vi "pulse Tx 8 spc.vi"(8 "clear DDS":bool, 9 "enable line":bool=TRUE, 10 "take it!":bool, 11 "Cluster":T2={"PW"=0, "frequency shift"=0.0, "amp"=0.9999923706054688, "mode type"=enum."CW", "mode depth"=0, "mode filter"=0, "phase shift"=0.0, "pulse shape filter"=0, "sub spc delay"=0}) -> (0 "output valid":bool, 1 "IQ out":T1[](array[typedef]), 2 "free dds":bool, 4 "frequncy":fxp<+/-,48,0>, 6 "phase":fxp<+/-,16,1>)   [LabVIEW 2021]
uses:
  pulse_tx_vis/pdw.ctl
  pulse_tx_vis/CTL/mode_type.ctl
  <instrlib>/_niInstr/DSP/v1/Shared/Public/IQ Data.ctl
  <instrlib>/_niInstr/DSP/v1/FPGA/Public/Sub VIs/Frequency Shift/Frequency Shift - 8 spc.vi
  <instrlib>/_niInstr/Basic Elements/v1/FPGA/Private/Count Up U32.vi
  <vilib>/rvi/FXPMathLib/FxpAdd/XNode/nifxpmath_Add.xnode
  <instrlib>/_niInstr/DSP/v1/Shared/niInstr DSP v1 Shared.lvlib
  <instrlib>/_niInstr/Basic Elements/v1/FPGA/niInstr Basic Elements v1 FPGA.lvlib
  <vilib>/rvi/FXPMathLib/sim/FxpSim.dll
  <instrlib>/_niInstr/DSP/v1/FPGA/niInstr DSP v1 FPGA.lvlib
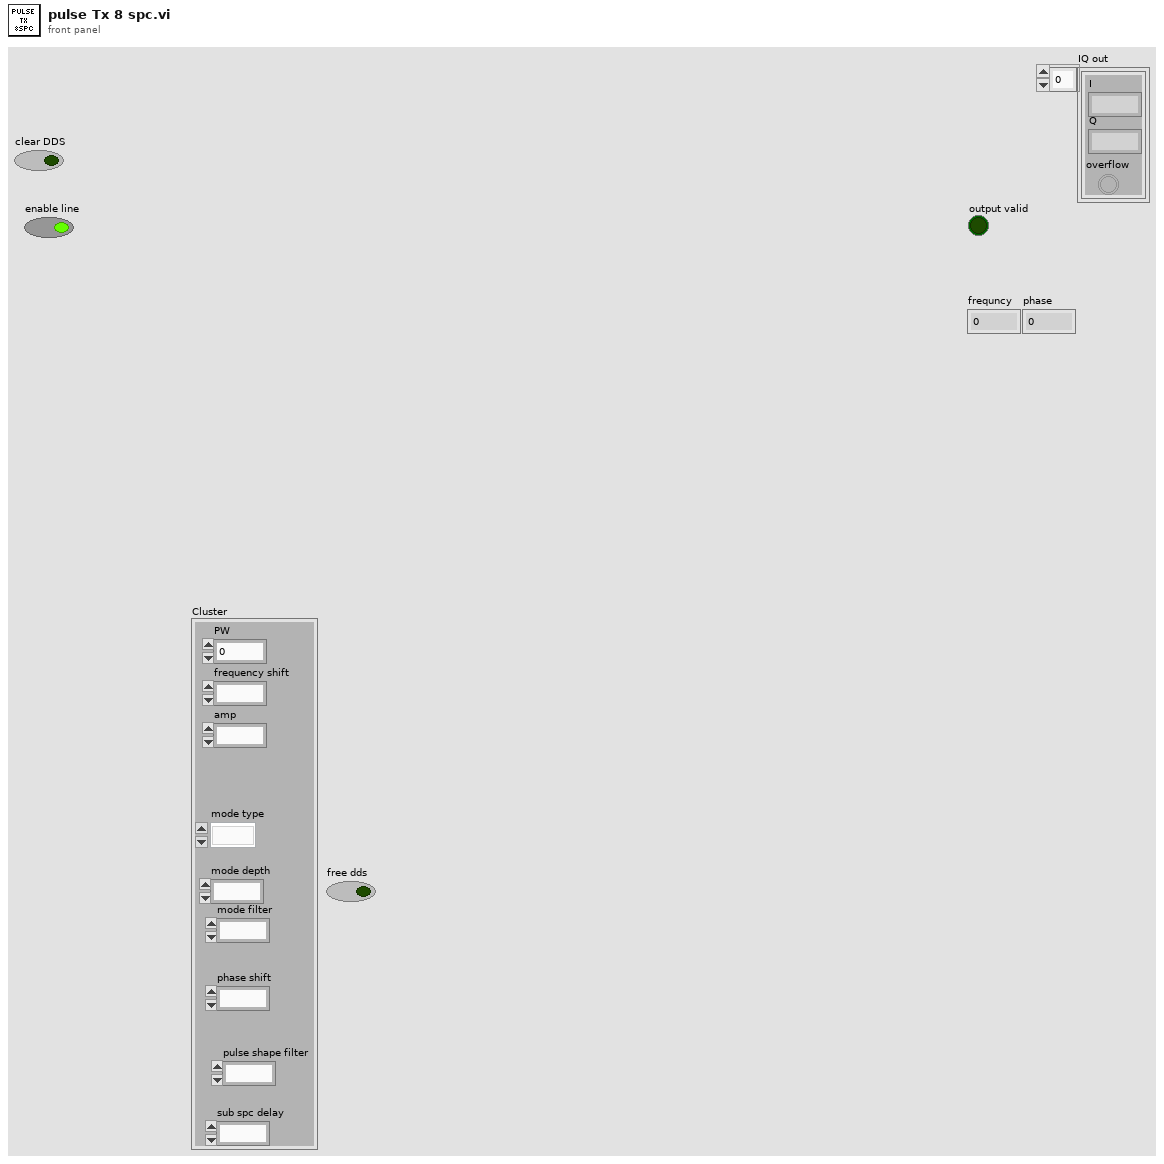
[diagram p1: front panel]
types:
  T1 = typedef "niInstr DSP v1 Shared.lvlib/IQ Data.ctl" = cluster{"I":fxp<+/-,18,1>, "Q":fxp<+/-,18,1>, "overflow":bool}
  T2 = typedef "pdw.ctl" = cluster{"PW":u32, "frequency shift":fxp<+/-,48,0>, "amp":fxp<+/-,18,1>, "mode type":T3, "mode depth":u32, "mode filter":u8, "phase shift":fxp<+/-,16,1>, "pulse shape filter":u8, "sub spc delay":u8}
  T3 = typedef "mode_type.ctl" = enum8{"CW", "from memory 1", "NC - cw", "LFM", "BPSK", "QPSK"}
  T4 = cluster{"I":fxp<+/-,18,1>, "Q":fxp<+/-,18,1>, "overflow":bool}[]
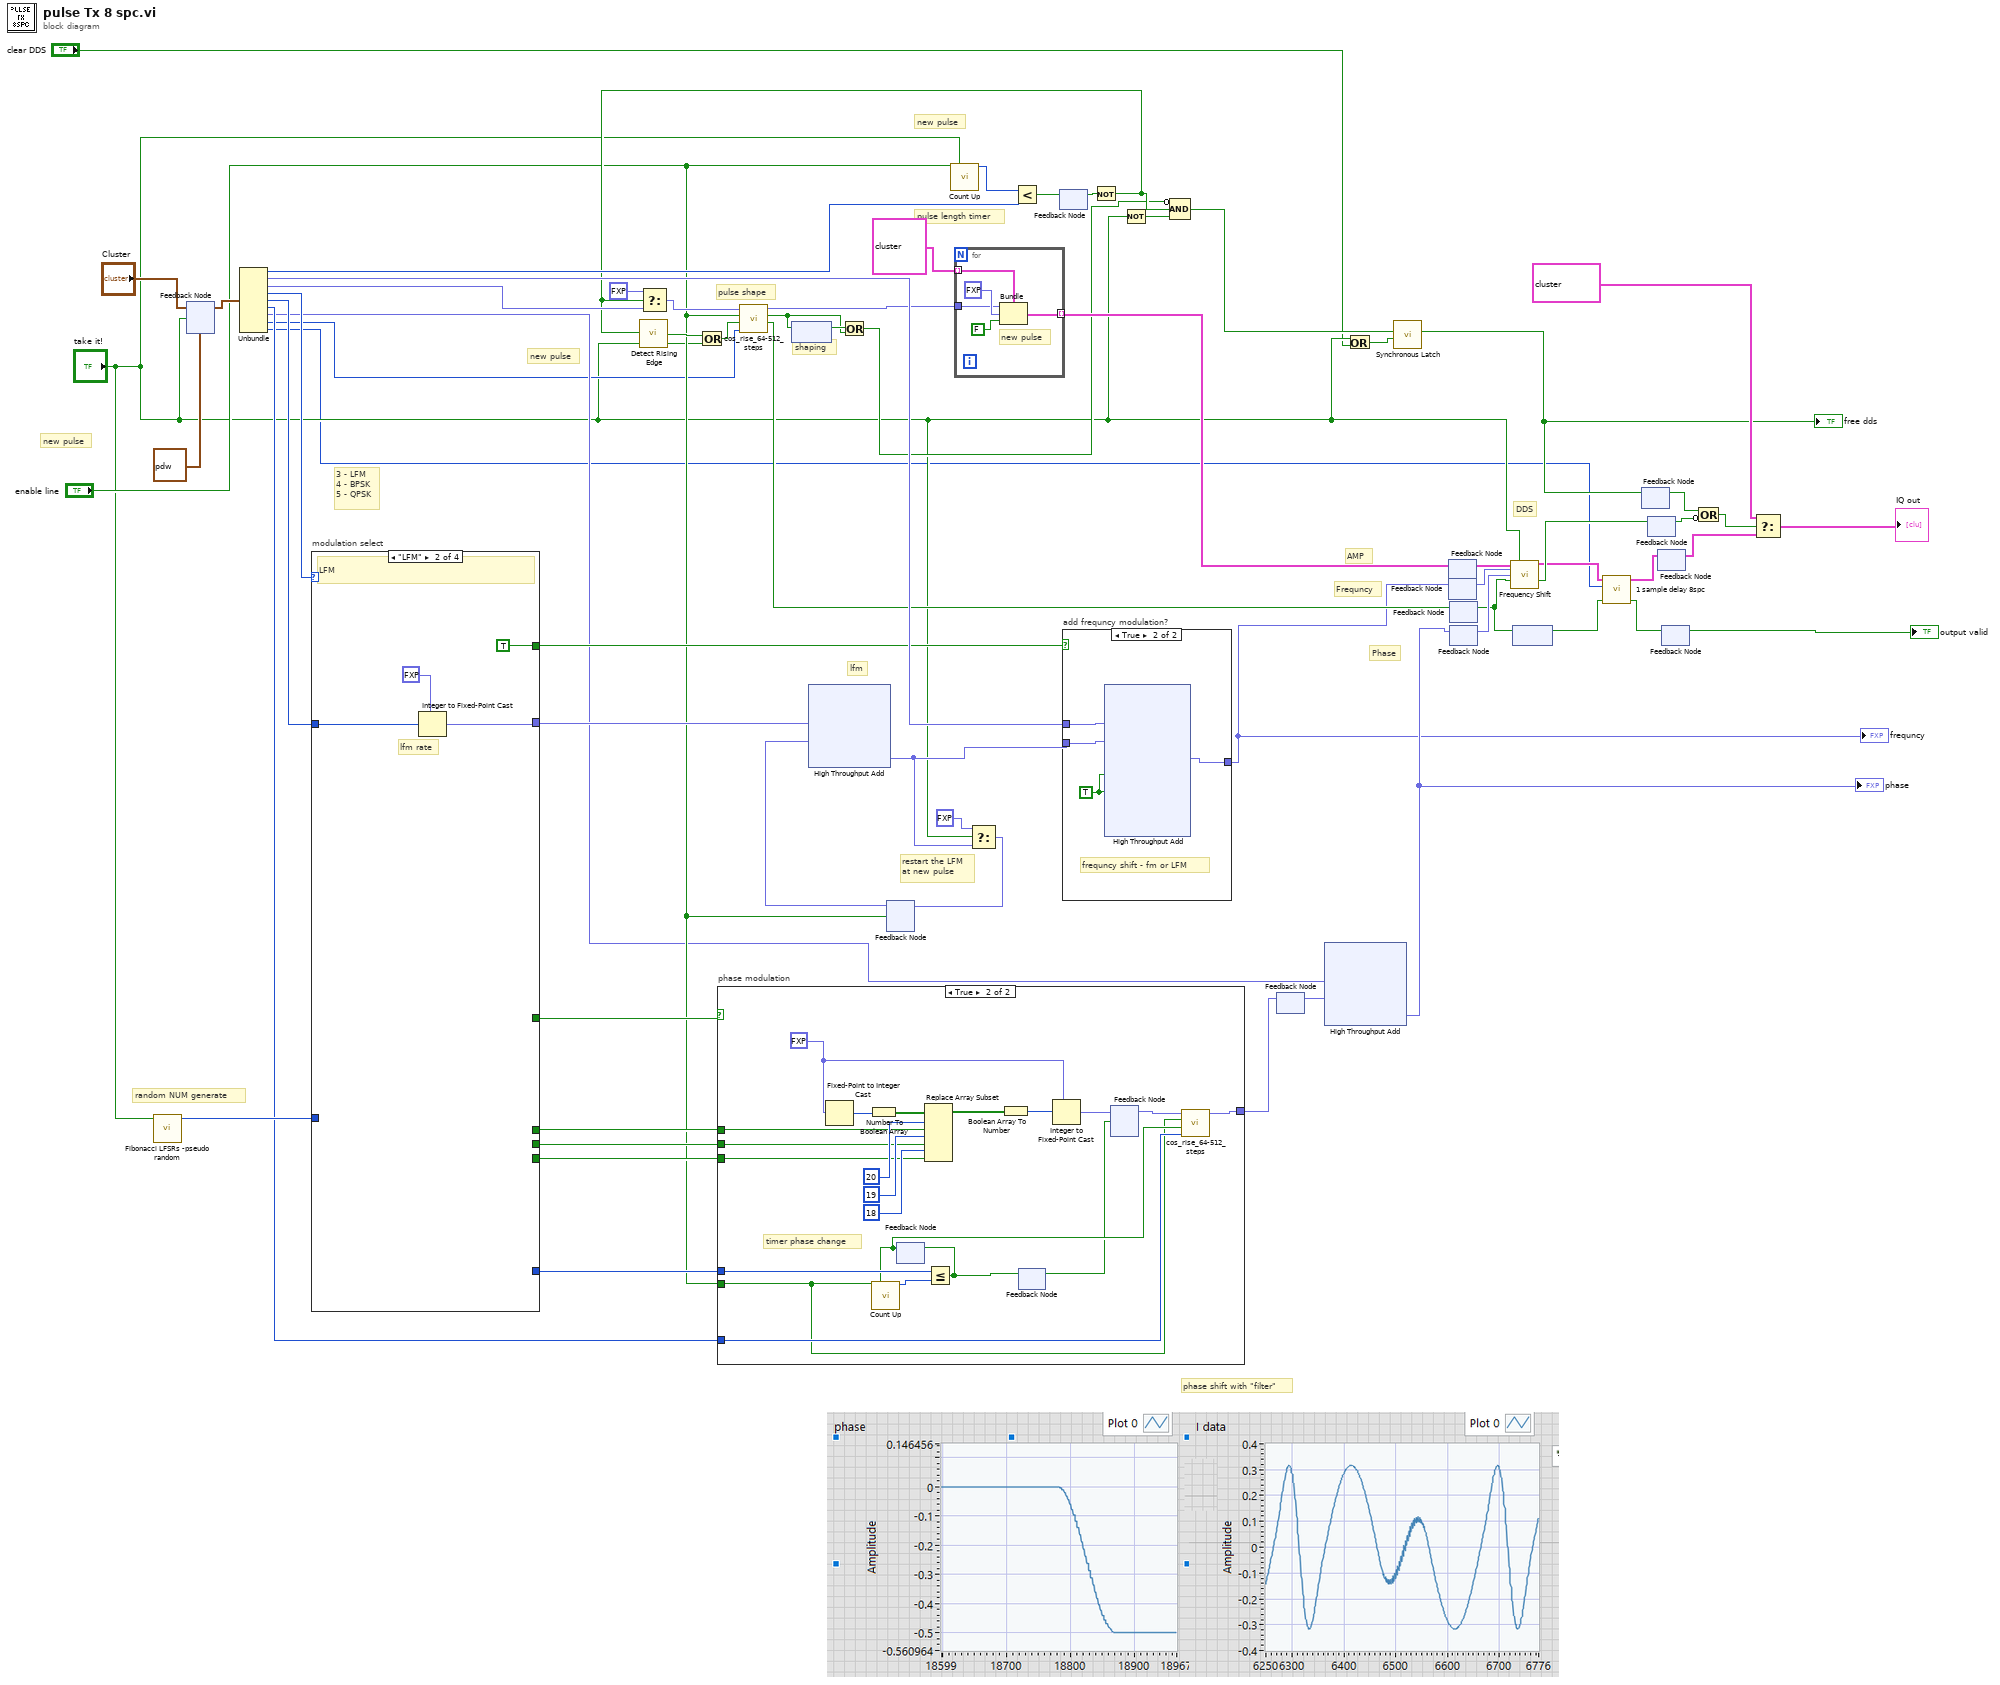
[diagram p0: block diagram]
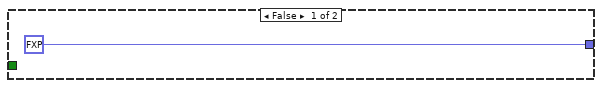
[diagram p2: hidden frame]
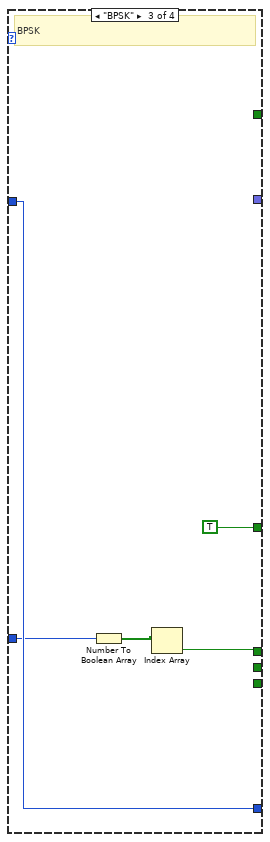
[diagram p5: hidden frame]
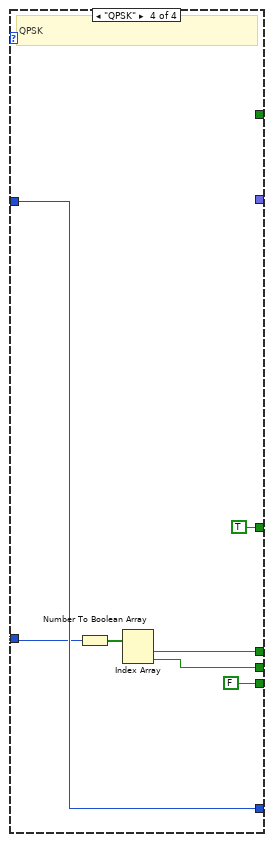
[diagram p6: hidden frame]
diagram:
  # "random NUM generate"
  # "phase shift with \"filter\""
  # "Phase"
  # "Frequncy"
  # "AMP"
  # "DDS"
  # "shaping"
  # "3 - LFM\n4 - BPSK\n5 - QPSK"
  # "pulse length timer"
  # "restart the LFM\nat new pulse"
  # "lfm"
  # "pulse shape"
  # "new pulse"
  # "new pulse"
  # "new pulse"
  n1 = call "Fibonacci LFSRs -pseudo random.vi"("reset random"="take it!") -> ("rand number"=w41:u16)  [unwired: 10 in]
  n2 = feedback #1(T2 {"PW"=0, "frequency shift"=0.0, "amp"=0.9999923706054688, "mode type"=enum."CW", "mode depth"=0, "mode filter"=0, "phase shift"=0.0, "pulse shape filter"=0, "sub spc delay"=0} ("Cluster")) -> (w64:T2)
  n3 = feedback-in #1("Cluster", "take it!") -> ()
  n4 = Unbundle(w64) -> ("PW"=w66:u32, "frequency shift"=w60:fxp<+/-,48,0>, "amp"=w44:fxp<+/-,18,1>, "mode type"=w61:T3, "mode depth"=w36:u32, "mode filter"=w35:u8, "phase shift"=w33:fxp<+/-,16,1>, "pulse shape filter"=w20:u8, "sub spc delay"=w1:u8)
  n5 = case "modulation select" shown="\"LFM\"" w61 {
    tunnel: w36 -> [_ w69 w72 w77]
    tunnel: [_ w68 _ _] -> w57
    tunnel: [_ TRUE ("s") _ _] -> w54
    tunnel: [_ _ _ FALSE] -> w52
    tunnel: [_ _ _ w79] -> w51
    tunnel: [_ _ w74 w81] -> w50
    tunnel: [_ _ TRUE TRUE] -> w49
    tunnel: [_ _ w72 w77] -> w48
    tunnel: w41 -> [_ _ w71 w76]
    frame Default {
    }
    frame "LFM" {
      # "lfm rate"
      # "LFM"
      n6 = Integer to Fixed-Point Cast(fixed-point type=fxp<+/-,32,-16> 0.0, integer=w69) -> (fixed-point=w68:fxp<+/-,32,-16>)
    }
    frame "BPSK" {
      # "BPSK"
      n7 = Number To Boolean Array(number=w71) -> (Boolean array=w75:bool[])
      n8 = Index Array(array=w75) -> (element=w74:bool)  [unwired: 1 in]
    }
    frame "QPSK" {
      # "QPSK"
      n9 = Number To Boolean Array(number=w76) -> (Boolean array=w82:bool[])
      n10 = Index Array(array=w82) -> (element #1=w81:bool, element #2=w79:bool)  [unwired: 2 in]
    }
  }
  n11 = case "phase modulation" shown="True" w49 {
    tunnel: w52 -> [_ w96]
    tunnel: w51 -> [_ w95]
    tunnel: w50 -> [_ w94]
    tunnel: w48 -> [_ w92]
    tunnel: [fxp<+/-,16,1> 0.0 ("filter out") w89] -> w22
    tunnel: w35 -> [_ w87]
    tunnel: "enable line" -> [_ w86]
    frame False {
    }
    frame True {
      w98 = fxp<+/-,21,0> 0.0 ("phase")
      # "timer phase change"
      n12 = Fixed-Point to Integer Cast(1:w98) -> (0:w104:i32)
      n13 = Number To Boolean Array(number=w104) -> (Boolean array=w102:bool[])
      n14 = feedback #2() -> (w88:bool)  [unwired: 1 in]
      n15 = call-poly <instrlib>:"Count Up.vi"("increment"=w86, "reset"=w88) -> ("count out"=w91:u32)  [unwired: 13 in]
      n16 = Replace Array Subset(array=w102, new element #1=w94, index #1=20 ("index"), new element #2=w95, index #2=19 ("index"), new element #3=w96, index #3=18 ("index")) -> (w97:bool[])
      n17 = Less Or Equal?(x=w92, y=w91) -> (x <= y?=w85:bool)
      n18 = feedback-in #2(w85) -> ()
      n19 = Boolean Array To Number(Boolean array=w97) -> (number=w103:u32)
      n20 = feedback-in #3(w85) -> ()
      n21 = feedback #3() -> (w84:bool)  [unwired: 1 in]
      n22 = Integer to Fixed-Point Cast(fixed-point type=w98, integer=w103) -> (fixed-point=w93:fxp<+/-,21,0>)
      n23 = feedback-in #4(w93, w84) -> ()
      n24 = feedback #4() -> (w90:fxp<+/-,21,0>)  [unwired: 1 in]
      n25 = call "cos_rise_64-512_steps.vi"("filter select"=w87, "new step"=w88, "run"=w86, "data in"=w90) -> ("data out"=w89:fxp<+/-,16,1>)  [unwired: 5 in, 2 out]
    }
  }
  n26 = feedback #5() -> (w12:bool)  [unwired: 1 in]
  n27 = feedback #6() -> (w56:fxp<+/-,48,0>)  [unwired: 1 in]
  n28 = xnode ("High Throughput Add")("x"=w57, "y"=w56) -> ("x+y"=w55:fxp<+/-,48,0>)
  n29 = call-poly <instrlib>:"Count Up.vi"("increment"="enable line", "reset"="take it!") -> ("count out"=w47:u32)  [unwired: 13 in]
  n30 = Select(t=fxp<+/-,48,0> 0.0, s="take it!", f=w55) -> (s? t:f=w58:fxp<+/-,48,0>)
  n31 = feedback-in #6(w58, "enable line") -> ()
  n32 = Less?(x=w47, y=w66) -> (x < y?=w46:bool)
  n33 = feedback #7() -> (w45:bool)  [unwired: 1 in]
  n34 = feedback-in #7(w46) -> ()
  n35 = case "add frequncy modulation?" shown="True" w54 {
    tunnel: w60 -> [w105 w109]
    tunnel: w55 -> [_ w108]
    tunnel: [w105 w107] -> w30
    frame False {
    }
    frame True {
      w106 = TRUE ("input valid")
      # "frequncy shift - fm or LFM"
      n36 = xnode ("High Throughput Add")("x"=w109, "y"=w108, "input valid"=w106, "ready for output (T)"=w106) -> ("x+y"=w107:fxp<+/-,48,0>)  [unwired: 2 out]
    }
  }
  "frequncy" <- w30
  n37 = Not(x=w45) -> (.not. x?=w38:bool)
  n38 = call <instrlib>:"Detect Rising Edge.vi"("signal"=w38) -> ("edge detected"=w37:bool)  [unwired: 14 in]
  n39 = Select(t=fxp<+/-,18,1> 0.0, s=w38, f=w44) -> (s? t:f=w43:fxp<+/-,18,1>)
  n40 = Or(x=w37, y="take it!") -> (x .or. y?=w39:bool)
  n41 = call "cos_rise_64-512_steps.vi"("filter select"=w20, "new step"=w39, "run"="enable line", "data in"=w43) -> ("output valid"=w31:bool, "steping"=w11:bool, "data out"=w40:fxp<+/-,16,1>)  [unwired: 5 in]
  n42 = feedback-in #5(w11) -> ()
  n43 = Or(x=w12, y=w11) -> (x .or. y?=w10:bool)
  n44 = for {
    tunnel: w40 -> [w112]
    tunnel: [w111] -> w29 mode=indexing
    tunnel: T1[] [{"I"=0.0, "Q"=0.0, "overflow"=FALSE}, {"I"=0.0, "Q"=0.0, "overflow"=FALSE}, {"I"=0.0, "Q"=0.0, "overflow"=FALSE}, {"I"=0.0, "Q"=0.0, "overflow"=FALSE}, {"I"=0.0, "Q"=0.0, "overflow"=FALSE}, {"I"=0.0, "Q"=0.0, "overflow"=FALSE}, {"I"=0.0, "Q"=0.0, "overflow"=FALSE}, {"I"=0.0, "Q"=0.0, "overflow"=FALSE}] ("t") -> [w110] mode=indexing
    # "new pulse"
    n45 = Bundle(cluster=w110, "I"=w112, "Q"=fxp<+/-,18,1> 0.0, "overflow"=FALSE ("input valid")) -> (w111:T1)
  }
  n46 = Not(x="take it!") -> (.not. x?=w63:bool)
  n47 = Compound Arithmetic op=AND(invert w10, w38, w63) -> (w62:bool)
  n48 = feedback-in #8(w22) -> ()
  n49 = feedback #8() -> (w21:fxp<+/-,16,1>)  [unwired: 1 in]
  n50 = xnode ("High Throughput Add")("x"=w33, "y"=w21) -> ("x+y"=w32:fxp<+/-,16,1>)
  "phase" <- w32
  n51 = Or(x="take it!", y="clear DDS") -> (x .or. y?=w8:bool)
  n52 = call <instrlib>:"Synchronous Latch.vi"("clear"=w8, "set"=w62) -> ("out"=w14:bool)  [unwired: 9 in]
  "free dds" <- w14
  n53 = feedback #9() -> (w24:T1[])  [unwired: 1 in]
  n54 = feedback-in #9(w29) -> ()
  n55 = feedback #10() -> (w28:fxp<+/-,48,0>)  [unwired: 1 in]
  n56 = feedback-in #10(w30) -> ()
  n57 = feedback #11() -> (w17:bool)  [unwired: 1 in]
  n58 = feedback-in #11(w31) -> ()
  n59 = feedback-in #12(w32) -> ()
  n60 = feedback #12() -> (w27:fxp<+/-,16,1>)  [unwired: 1 in]
  n61 = call-poly <instrlib>:"Frequency Shift.vi"("data in"=w24, "reset"="take it!", "frequency shift"=w28, "phase"=w27, "input valid"=w17) -> ("data out"=w5:T1[], "output valid"=w16:bool)  [unwired: 7 in, 2 out]
  n62 = feedback #13() -> (w3:bool)  [unwired: 1 in]
  n63 = feedback-in #13(w17) -> ()
  n64 = call "1 sample delay 8spc.vi"("input valid"=w3, "delay"=w1, "IQ in"=w5) -> ("output valid"=w2:bool, "IQ out"=w4:T4)  [unwired: 7 in]
  n65 = feedback #14() -> (w13:bool)  [unwired: 1 in]
  n66 = feedback-in #14(w14) -> ()
  n67 = feedback #15() -> (w15:bool)  [unwired: 1 in]
  n68 = feedback-in #15(w16) -> ()
  n69 = feedback #16() -> (w23:T4)  [unwired: 1 in]
  n70 = feedback-in #16(w4) -> ()
  n71 = feedback #17() -> (→"output valid":bool)  [unwired: 1 in]
  n72 = feedback-in #17(w2) -> ()
  n73 = Compound Arithmetic op=OR(w13, invert w15) -> (w19:bool)
  n74 = Select(t=T1[] [{"I"=0.0, "Q"=0.0, "overflow"=FALSE}, {"I"=0.0, "Q"=0.0, "overflow"=FALSE}, {"I"=0.0, "Q"=0.0, "overflow"=FALSE}, {"I"=0.0, "Q"=0.0, "overflow"=FALSE}, {"I"=0.0, "Q"=0.0, "overflow"=FALSE}, {"I"=0.0, "Q"=0.0, "overflow"=FALSE}, {"I"=0.0, "Q"=0.0, "overflow"=FALSE}, {"I"=0.0, "Q"=0.0, "overflow"=FALSE}], s=w19, f=w23) -> (s? t:f=→"IQ out":T1[])
